vi "find all instances with alias.vi"(11 "flat hierarchy":T2) -> (3 "instance data":T1[](array[typedef]))   [LabVIEW 2013, in "NISE_CEF_TreeSerializer.lvlib"]
uses:
  NISE_CEF_TreeSerializer.lvlib
  flat hierarchy.ctl
  full hierarchy.ctl
  hierarchy element.ctl
  instance data.ctl
panel:
  in  "Alias":string
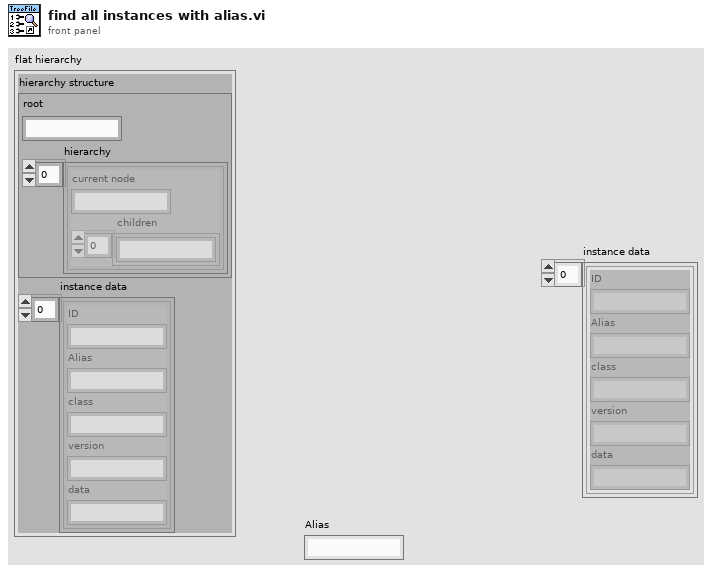
[diagram p1: front panel]
types:
  T1 = typedef "NISE_CEF_TreeSerializer.lvlib/instance data.ctl" = cluster{"ID":string, "Alias":string, "class":string, "version":string, "data":string}
  T2 = typedef "NISE_CEF_TreeSerializer.lvlib/flat hierarchy.ctl" = cluster{"hierarchy structure":T3, "instance data":T1[]}
  T3 = typedef "NISE_CEF_TreeSerializer.lvlib/full hierarchy.ctl" = cluster{"root":string, "hierarchy":T4[]}
  T4 = typedef "NISE_CEF_TreeSerializer.lvlib/hierarchy element.ctl" = cluster{"current node":string, "children":string[]}
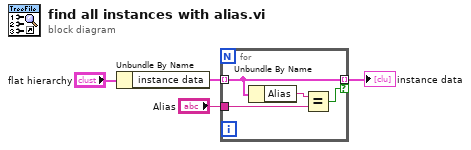
[diagram p0: block diagram]
diagram:
  n1 = Unbundle By Name("flat hierarchy") -> ("instance data"=w3:T1[])
  n2 = for {
    tunnel: w3 -> [w6] mode=indexing
    tunnel: "Alias" -> [w8]
    tunnel: [w6] -> w1 mode=indexing if=w5
    n3 = Unbundle By Name(w6) -> ("Alias"=w7:string)
    n4 = Equal?(x=w7, y=w8) -> (x = y?=w5:bool)
  }
  "instance data" <- w1
